vi "Send Start Polling.vi"(8 "error in (no error)":errorcluster, 11 "Message Queue in":refnum<queue>) -> (0 "error out":errorcluster, 3 "Message Queue out":refnum<queue>)   [LabVIEW 2024, in "OOQMH.lvlib" / "Start Polling.lvclass"]
uses:
  Start Polling.lvclass
  Start Polling.lvclass/Start Polling.ctl
  C:/Users/uspoaotto/OneDrive - Oregon Tool/Desktop/working copies/helperLoop/src/OOQMH/Message/Message.lvclass
  C:/Users/uspoaotto/OneDrive - Oregon Tool/Desktop/working copies/helperLoop/src/OOQMH/Start Polling/Start Polling.lvclass
  Message/Message.lvclass
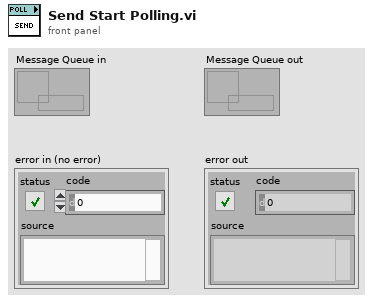
[diagram p1: front panel]
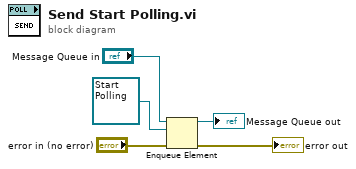
[diagram p0: block diagram]
diagram:
  n1 = Enqueue Element(queue="Message Queue in", element=refnum<class "Start Polling.lvclass"> refnum ("OOQMH.lvlib:Start Polling.lvclass"), error in (no error)="error in (no error)") -> (queue out=→"Message Queue out":refnum<queue>, error out=→"error out":errorcluster)  [unwired: 1 in, 1 out]
